vi "Clean href.vi"(11 "html in":string="sdfsfsse") -> (0 "after hyperlink":string, 1 "text":string, 2 "link":string, 3 "before hyperlink":string, 4 "Success?":bool)   [LabVIEW 2020]
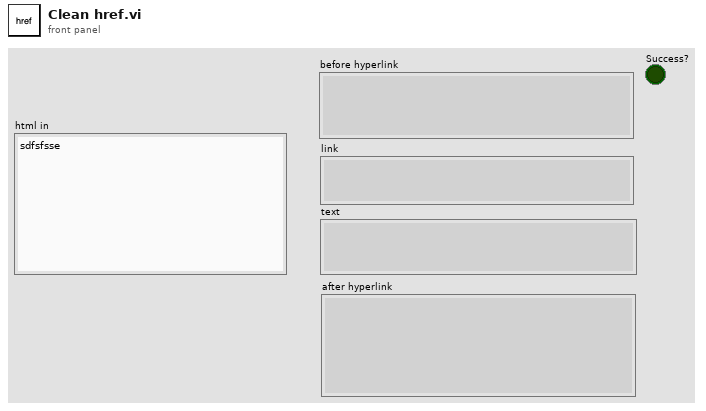
[diagram p1: front panel]
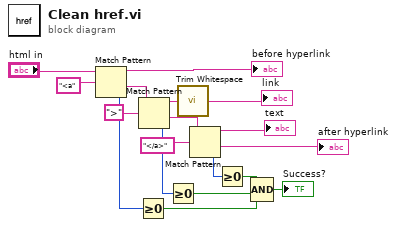
[diagram p0: block diagram]
diagram:
  n1 = Match Pattern(string="html in", regular expression="<a" ("format string")) -> (before substring=→"before hyperlink":string, after substring=w16:string, offset past match=w7:i32)  [unwired: 1 in, 1 out]
  n2 = Greater Or Equal To 0?(x=w7) -> (x >= 0?=w2:bool)
  n3 = Match Pattern(string=w16, regular expression=">" ("format string")) -> (before substring=w11:string, after substring=w13:string, offset past match=w6:i32)  [unwired: 1 in, 1 out]
  n4 = Greater Or Equal To 0?(x=w6) -> (x >= 0?=w3:bool)
  n5 = call <vilib>:"Trim Whitespace.vi"("string"=w11) -> ("trimmed string"=→"link":string)  [unwired: 1 in]
  n6 = Match Pattern(string=w13, regular expression="</a>" ("format string")) -> (before substring=→"text":string, after substring=→"after hyperlink":string, offset past match=w5:i32)  [unwired: 1 in, 1 out]
  n7 = Greater Or Equal To 0?(x=w5) -> (x >= 0?=w4:bool)
  n8 = Compound Arithmetic op=AND(w4, w3, w2) -> (→"Success?":bool)
